vi "create standard response header.vi"() -> (3 "default header":T1)   [LabVIEW 2016, in "https responder.lvclass"]
uses:
  https responder.lvclass
  HTTP headers/http header data.ctl
  HTTP headers/http headers.lvlib
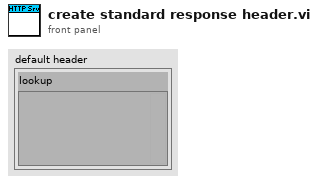
[diagram p1: front panel]
types:
  T1 = typedef "http headers.lvlib/http header data.ctl" = cluster{"lookup":variant}
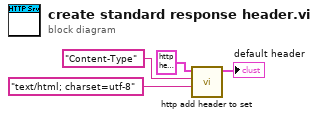
[diagram p0: block diagram]
diagram:
  n1 = call "http add header to set.vi"("header field data"="text/html; charset=utf-8" ("name"), "header field name"="Content-Type" ("name"), "headers in"=T1 {"lookup"=variant}) -> ("headers out"=→"default header":T1)  [unwired: 8 in]
